vi "svl_Add New Events.vi"(3 "New Events":bool[](array[boolean]), 4 "Event Names":string[](array[string]), 5 "Event Queue In":string[](array[string])) -> (2 "Event Queue Out":string[](array[string]))   [LabVIEW 2017]
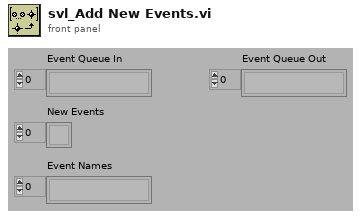
[diagram p1: front panel]
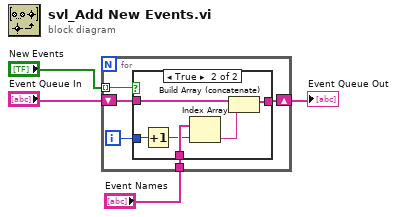
[diagram p0: block diagram]
diagram:
  n1 = for {
    shift-right: [w7] -> w1
    shift-left: "Event Queue In" -> [w8]
    tunnel: "New Events" -> [w6] mode=indexing
    tunnel: "Event Names" -> [w5]
    i -> [w9]
    n2 = case shown="True" w6 {
      tunnel: w9 -> [_ w12]
      tunnel: w8 -> [w10 w16]
      tunnel: [w10 w15] -> w7
      tunnel: w5 -> [_ w13]
      frame False {
      }
      frame True {
        n3 = Increment(x=w12) -> (x+1=w11:i32)
        n4 = Index Array(array=w13, index=w11) -> (element=w14:string)
        n5 = Build Array (concatenate)(w16, w14) -> (w15:string[])
      }
    }
  }
  "Event Queue Out" <- w1
